vi "gearGrabber.vi"(9 "gearStatus":bool, 11 "gear":string="My Servo RefNum") -> (0 "error out":errorcluster)   [LabVIEW 2016]
uses:
  <vilib>/Rock Robotics/WPI/Solenoid/WPI_SolenoidValue.ctl
  <vilib>/Rock Robotics/WPI/Solenoid/WPI_SolenoidSetEnum.vi
panel:
  in  "error in (no error)":errorcluster
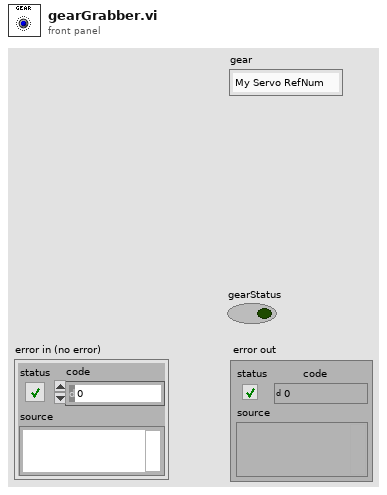
[diagram p1: front panel]
types:
  T1 = typedef "WPI_SolenoidDevRef.ctl" = cluster{"DevStatus":errorcluster, "Pneumatics Control Module":u8, "Forward Solenoid Channel":T2, "Reverse Solenoid Channel":T2}
  T2 = typedef "WPI_SolenoidChannel.ctl" = enum8{"Solenoid 0", "Solenoid 1", "Solenoid 2", "Solenoid 3", "Solenoid 4", "Solenoid 5", "Solenoid 6", "Solenoid 7", "Invalid"}
  T3 = typedef "WPI_SolenoidValue.ctl" = enum16{"Off", "On", "Forward", "Reverse"}
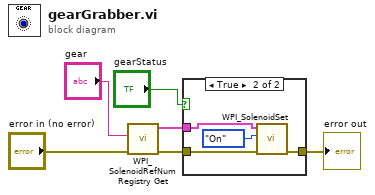
[diagram p0: block diagram]
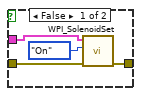
[diagram p2: hidden frame]
diagram:
  n1 = call <vilib>:"WPI_SolenoidRefNum Registry Get.vi"("error in (no error)"="error in (no error)", "refnum name"="gear") -> ("error out"=w1:errorcluster, "SolenoidDevRef"=w4:T1)  [unwired: 8 in]
  n2 = case shown="True" "gearStatus" {
    tunnel: w4 -> [w9 w13]
    tunnel: [w7 w11] -> w5
    tunnel: w1 -> [w8 w12]
    frame False {
      n3 = call-poly <vilib>:"WPI_SolenoidSet.vi"("error in (no error)"=w8, "Value"=WPI_SolenoidValue."On", "SolenoidDevRef"=w9) -> ("error out"=w7:errorcluster)  [unwired: 7 in, 1 out]
    }
    frame True {
      n4 = call-poly <vilib>:"WPI_SolenoidSet.vi"("error in (no error)"=w12, "Value"=WPI_SolenoidValue."On", "SolenoidDevRef"=w13) -> ("error out"=w11:errorcluster)  [unwired: 7 in, 1 out]
    }
  }
  "error out" <- w5
